vi "Measure (Poly).vi"   [LabVIEW 2014, in "niHighSpeedSerial Eye Scan v1 Host.lvclass"]
doc: "Returns points that have been measured."
uses:
  <instrlib>/niHighSpeedSerial/Eye Scan/v1/Host/Eye Scan/niHighSpeedSerial Eye Scan v1 Host.lvclass
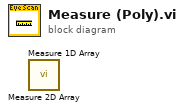
[diagram p0: block diagram]
diagram:
  n1 = call <instrlib>:"Measure 2D Array.vi"() -> ()  [unwired: 8 in, 8 out]
  n2 = call <instrlib>:"Measure 1D Array.vi"() -> ()  [unwired: 8 in, 8 out]
